vi "line driveable paths global.vi"() -> ()   [LabVIEW 2009]
uses:
  IO/vision serial/vision decoder state typedef.ctl
panel:
  out "DMA timeout":bool
  out "y data":i16
  out "x data":i16
  out "line driveable paths":u16[](array[numeric])
  out "scan number":u8
  out "decoder state":T1
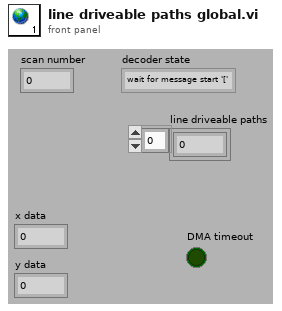
[diagram p1: front panel]
types:
  T1 = typedef "vision decoder state typedef.ctl" = enum16{"wait for message start '['", "wait for point start '(' ", "record x value", "record y value", "scan complete"}
diagram:
